vi "__UnpackNameMap.vi"(11 "Map":variant) -> (3 "NameMap":T1)   [LabVIEW 2019]
uses:
  Typedef/Def-NameMap.ctl
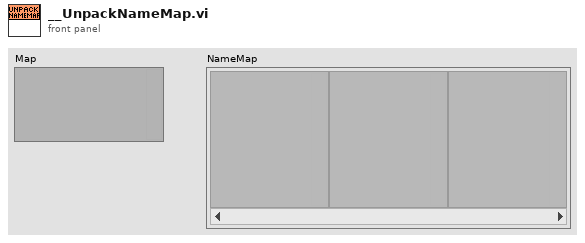
[diagram p1: front panel]
types:
  T1 = typedef "Def-NameMap.ctl" = variant[]
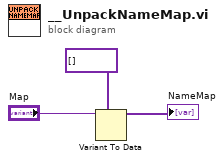
[diagram p0: block diagram]
diagram:
  n1 = Variant To Data(type=T1 [] ("AttrMap"), Variant="Map") -> (data=→"NameMap":T1)  [unwired: 1 in, 1 out]
